vi "set_piezos (SubVI).vi"(8 "error in":errorcluster, 10 "Tot Stage Arr":dbl[](array[numeric]), 11 "task/channels in":refnum<k21>) -> (0 "error out":errorcluster, 3 "task out":refnum<k21>)   [LabVIEW 2016]
uses:
  <vilib>/DAQmx/write.llb/DAQmx Write (Analog 1D DBL NChan 1Samp).vi
  <vilib>/DAQmx/miscellaneous.llb/DAQmx Fill In Error Info.vi
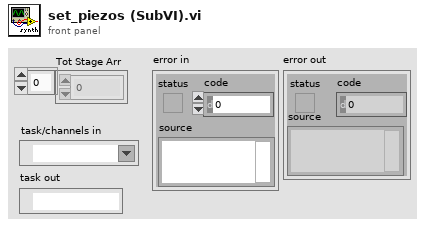
[diagram p1: front panel]
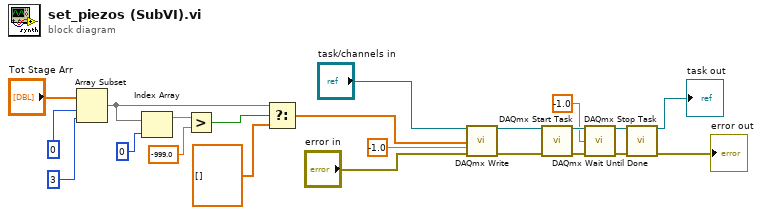
[diagram p0: block diagram]
diagram:
  n1 = Array Subset(array="Tot Stage Arr", index=0, length=3) -> (w6:dbl[])
  n2 = Index Array(array=w6, index=0) -> (element=w4:dbl)
  n3 = Greater?(x=w4, y=-999.0) -> (0:w2:bool)
  n4 = Select(t=w6, s=w2, f=dbl[] []) -> (s? t:f=w8:dbl[])
  n5 = call-poly <vilib>:"DAQmx Write.vi"("task/channels in"="task/channels in", "data"=w8, "timeout"=-1.0, "error in"="error in") -> ("task out"=w22:refnum<k21>, "error out"=w14:errorcluster)  [unwired: 9 in, 1 out]
  n6 = call <vilib>:"DAQmx Start Task.vi"("task/channels in"=w22, "error in"=w14) -> ("task out"=w21:refnum<k21>, "error out"=w15:errorcluster)  [unwired: 12 in]
  n7 = call <vilib>:"DAQmx Wait Until Done.vi"("task/channels in"=w21, "timeout (sec)"=-1.0, "error in"=w15) -> ("task out"=w20:refnum<k21>, "error out"=w16:errorcluster)  [unwired: 11 in]
  n8 = call <vilib>:"DAQmx Stop Task.vi"("task/channels in"=w20, "error in"=w16) -> ("task out"=→"task out":refnum<k21>, "error out"=→"error out":errorcluster)  [unwired: 12 in]
